vi "Send Message Normal Check.vi"(4 "Source (\"\")":string, 6 "Timeout (25000)":u32=25000, 8 "error in (no error)":errorcluster, 10 "Send Message (\"\")":string, 11 "VISA resource name":refnum<visa-resource-name>) -> (0 "error out":errorcluster, 1 "Read Buffer@":string, 2 "Response Type":i32(ring) items=["Affirmative", "Single Negative", "Multiple Negative", "ASCII", "Binary", "End"], 3 "VISA resource name out":refnum<visa-resource-name>, 5 "Internal Error Number":i32 max=999 step=1, 7 "Internal Error String":string)   [LabVIEW 2020, in "Yokogawa GX Series.lvlib"]
doc: "This VI sends the message. Then it returns the response and checks the message.\nThen this returns Internal Error Type. If the message is an error message, this sets \"command are not processed succesfully\" to error out."
uses:
  <instrlib>/Yokogawa GX Series/Yokogawa GX Series.lvlib
panel:
  # "msec"
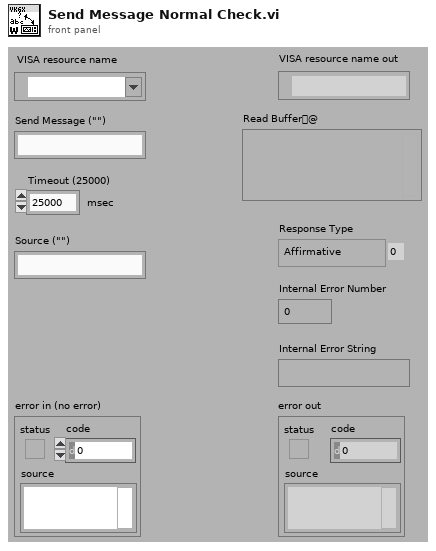
[diagram p1: front panel]
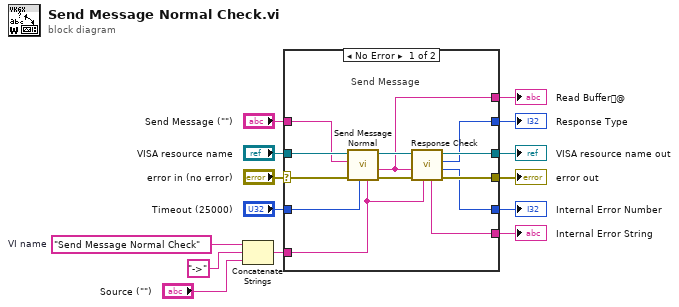
[diagram p0: block diagram]
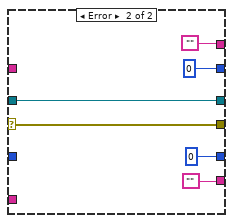
[diagram p2: hidden frame]
diagram:
  w14 = "Send Message Normal Check"  # VI name
  n1 = Concatenate Strings(w14, "->", "Source (\"\")") -> (w8:string)
  n2 = case shown="No Error" "error in (no error)" {
    selector: "error in (no error)" -> [w15 w30]
    tunnel: [w27 w31] -> w11
    tunnel: [w26 w30] -> w10
    tunnel: "VISA resource name" -> [w25 w31]
    tunnel: w8 -> [w22 _]
    tunnel: "Timeout (25000)" -> [w21 _]
    tunnel: "Send Message (\"\")" -> [w20 _]
    tunnel: [w19 0] -> w5
    tunnel: [w18 0] -> w4
    tunnel: [w17 ""] -> w3
    tunnel: [w16 ""] -> w2
    frame No Error {
      # "Send Message"
      n3 = call <instrlib>:"Send Message Normal.vi"("Source (\"\")"=w22, "Timeout (25000)"=w21, "error in (no error)"=w15, "Send Message (\"\")"=w20, "VISA resource name"=w25) -> ("error out"=w23:errorcluster, "Read Buffer"=w16:string, "VISA resource name out"=w24:refnum<visa-resource-name>)  [unwired: 4 out]
      n4 = call <instrlib>:"Response Check.vi"("Source (\"\")"=w22, "error in (no error)"=w23, "Message In (\"\")"=w16, "VISA resource name"=w24) -> ("error out"=w26:errorcluster, "Internal Error Number"=w18:i32, "Response Type"=w19:i32, "VISA resource name out"=w27:refnum<visa-resource-name>, "Internal Error String"=w17:string)  [unwired: 3 out]
    }
    frame Error {
    }
  }
  "error out" <- w10
  "VISA resource name out" <- w11
  "Internal Error Number" <- w4
  "Internal Error String" <- w3
  "Response Type" <- w5
  "Read Buffer@" <- w2
